vi "Process.vi"(8 "error in":errorcluster, 11 "Measurement.WavelengthSweeping.UI":refnum<class "Measurement.IVCurve.UI.lvclass">) -> (0 "error out":errorcluster, 3 "Measurement.WavelengthSweeping.UI out":refnum<class "Measurement.IVCurve.UI.lvclass">)   [LabVIEW 2017, in "Measurement.IVCurve.UI.lvclass"]
doc: "---------------------------------------------------------------\nJKI State Machine Objects™\nhttp://jki.net/state-machine-objects/\nCopyright (C) 2005-2015, JKI <info@jki.net>\nALL RIGHTS RESERVEDJKI State Machine Objects (SMO) 1.0.0.5\nJKI - JKI\nCopyright (c) 2016, JKI"
uses:
  Measurement.IVCurve.UI.lvclass
  D:/Program Files (x86)/National Instruments/LabVIEW 2017/vi.lib/JKI/JKI SMO/SMO/SMO.lvclass
  D:/Program Files (x86)/National Instruments/LabVIEW 2017/vi.lib/JKI/JKI SMO/SMO.UI/SMO.UI.lvclass
  <vilib>/JKI/JKI SMO/SMO/Typedefs/Parent Call--Enum.ctl
  Measurement.IVCurve/Typedefs/Measurement.IVCurve.Measured--Data.ctl
  Measurement.IVCurve/Measurement.IVCurve.lvclass
  D:/upwork/Laser Measurement Tool/Laser/project/Subsystems/Measurement/Measurement.lvclass
  Measurement.UI/Measurement.UI.lvclass
  <vilib>/JKI/JKI SMO/SMO/SMO.lvclass
  <vilib>/JKI/JKI SMO/SMO.UI/SMO.UI.lvclass
  Measurement/Measurement.lvclass
panel:
  in  "Clear Button":bool
  in  "Stop Button":bool
  in  "Pause Button":bool
  in  "Start Button":bool
  in  "Close Button":bool
  out "Initialized":bool
  out "I/V Curve":cluster{"X":dbl, "Y":dbl}[](graph) caption="XY Graph - Light"
  # "For instructions on how to use the JKI State Machine Objects, examples and video tutorials, visit:\nhttp://jki.net/state-machine-objects/\n\nJKI State Machine Objects™\nhttp://jki.net/state-machine-objects/\nCopyright (C) 2005-2015, JKI <info@jki.net>\nALL RIGHTS RESERVED"
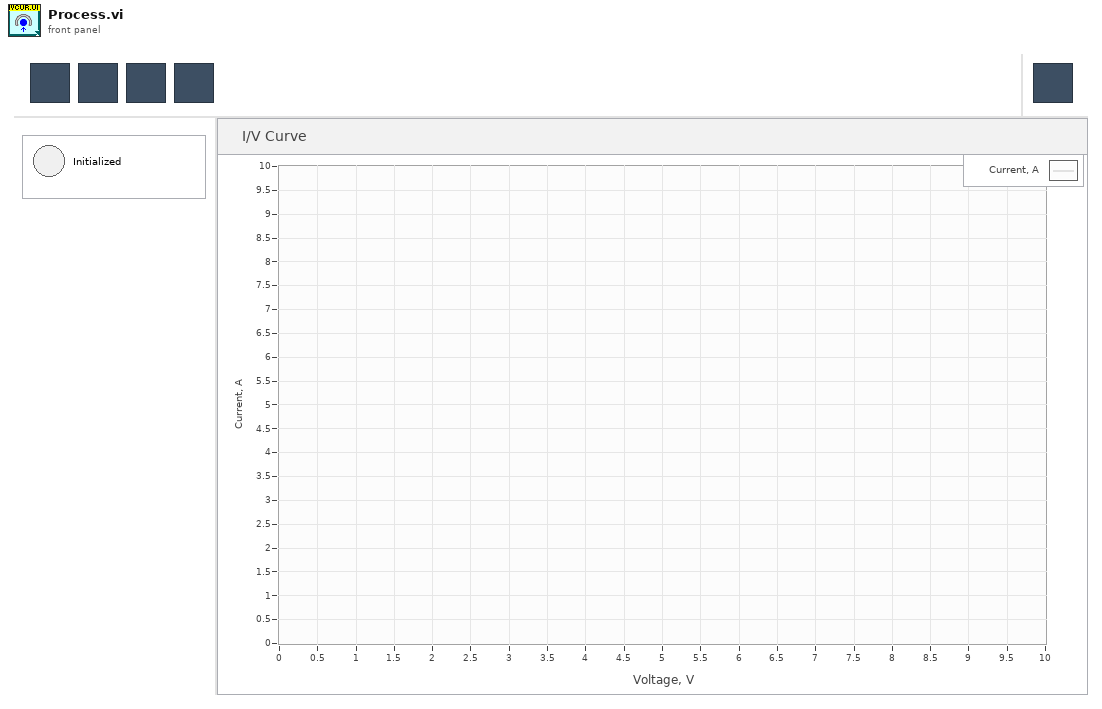
[diagram p1: front panel]
types:
  T1 = typedef "SMO.lvclass/Parent Call--Enum.ctl" = enum16{"Allows parent to run", "Does not request parent to run"}
  T2 = enum8{"Enabled", "Disabled", "Disabled and Grayed Out"}
  T3 = enum32{"invalid app kind", "Development System", "Run Time System", "Student Edition", "Embedded LabVIEW", "Evaluation", "Custom"}
  T4 = enum32{"Invalid", "Standard", "Closed", "Hidden", "Minimized", "Maximized"}
  T5 = typedef "Measurement.lvclass/PublicEvents--Measurement.Initialized.ctl" = bool
  T6 = typedef "Measurement.IVCurve.lvclass/Measurement.IVCurve.Measured--Data.ctl" = cluster{"Voltage, V":dbl, "Current, A":dbl}
  T7 = typedef "Measurement.lvclass/PublicEvents--Measurement.Measured.ctl" = variant
  T8 = typedef "Measurement.IVCurve.UI.lvclass/Dependencies--Cluster.ctl" = cluster{"Measurement.IVCurve":refnum<class "Measurement.IVCurve.lvclass">}
  T9 = cluster{"Core":cluster{"Current VI Reference":refnum<vi>, "Close Panel on Exit?":bool, "error":errorcluster}, "Self Reference":refnum<class "Measurement.IVCurve.UI.lvclass">, "Dependencies":T8, "IVCurve Data":cluster{"X":dbl, "Y":dbl}[]}
  T10 = typedef "Measurement.lvclass/PublicEvents--Measurement.Finished.ctl" = bool
  T11 = cluster{"Current VI Reference":refnum<vi>, "Close Panel on Exit?":bool, "error":errorcluster}
  T12 = typedef "SMO.lvclass/Protected Events.ctl" = cluster{"StopProcesses":refnum<user-event>, "AbortProcesses":refnum<user-event>, "Config Changed":refnum<user-event>, "Dependency":refnum<user-event>}
  T13 = cluster{"Event Registration Refnum":refnum<event-registration>, "Measurement Public Events":refnum<event-registration>}
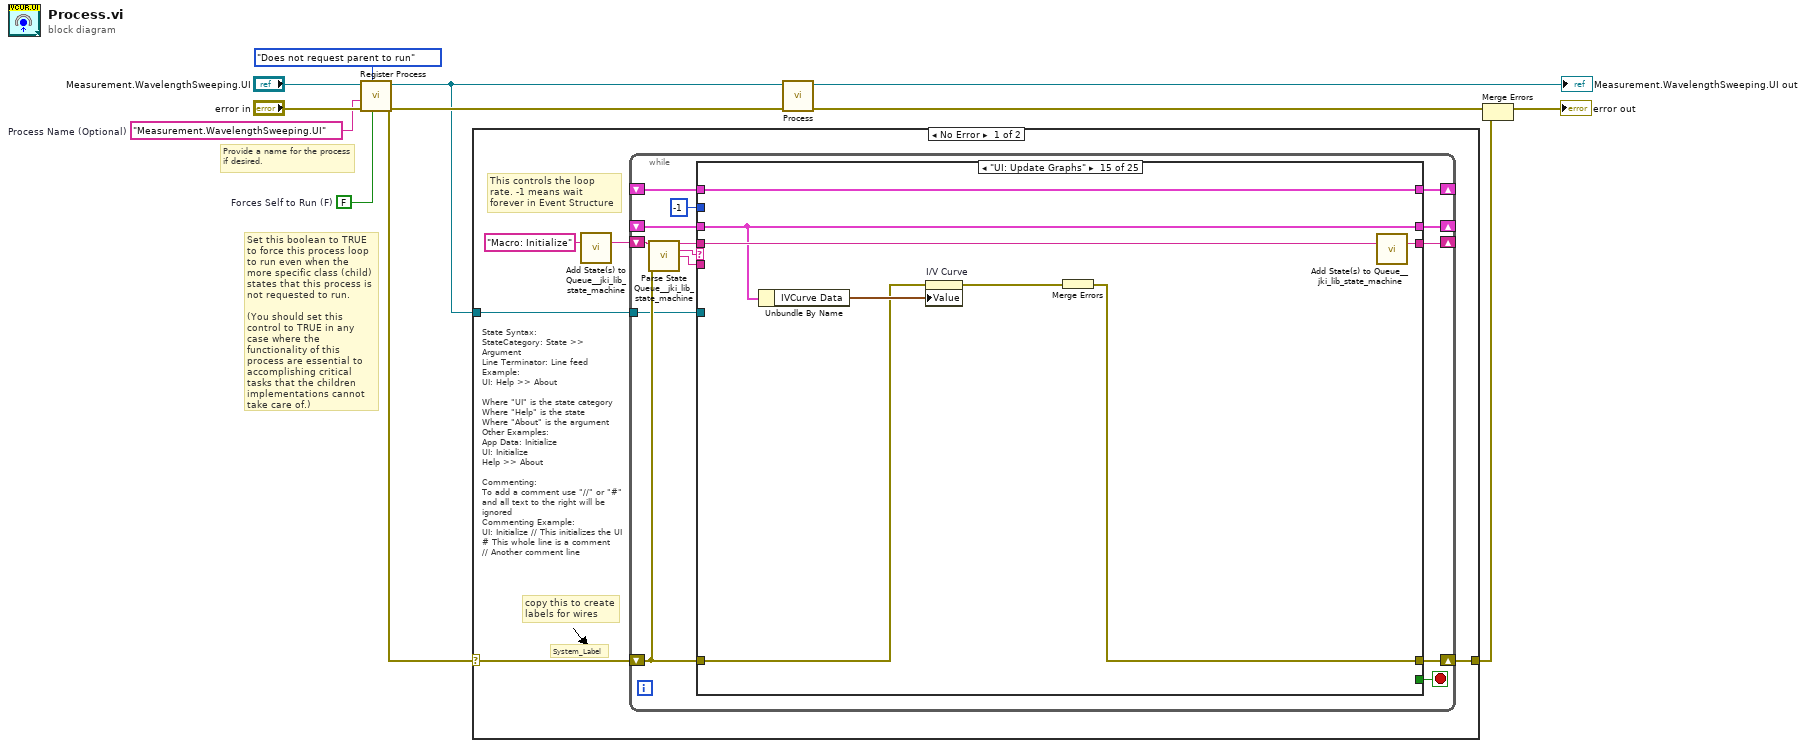
[diagram p0: block diagram]
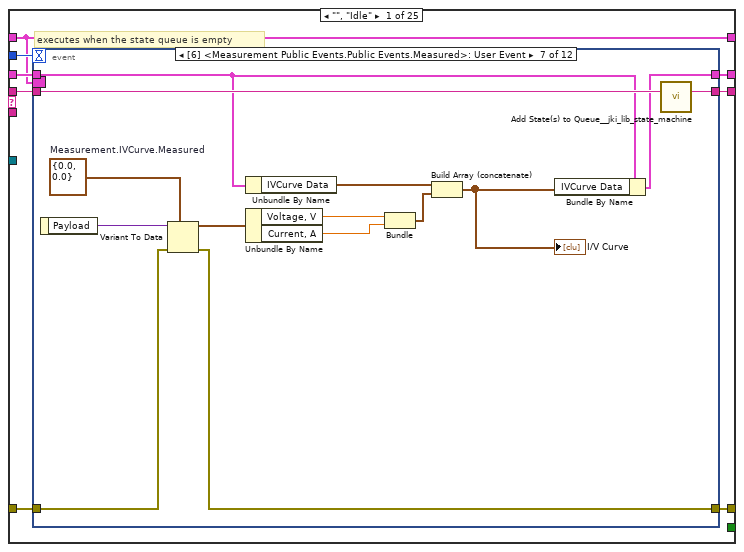
[diagram p2: hidden frame]
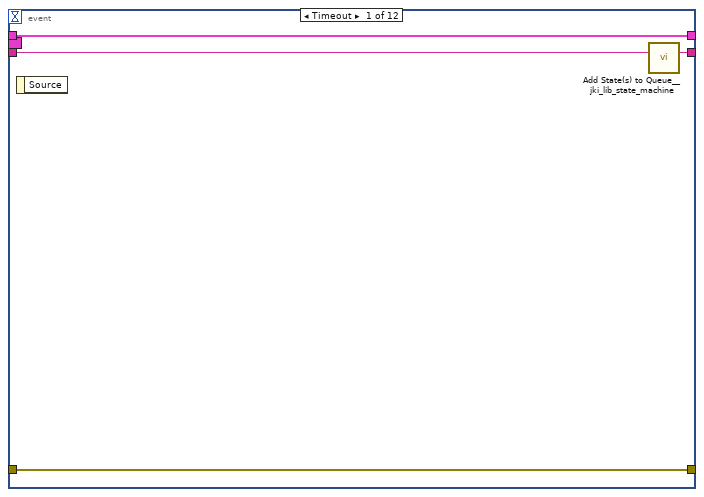
[diagram p3: hidden frame]
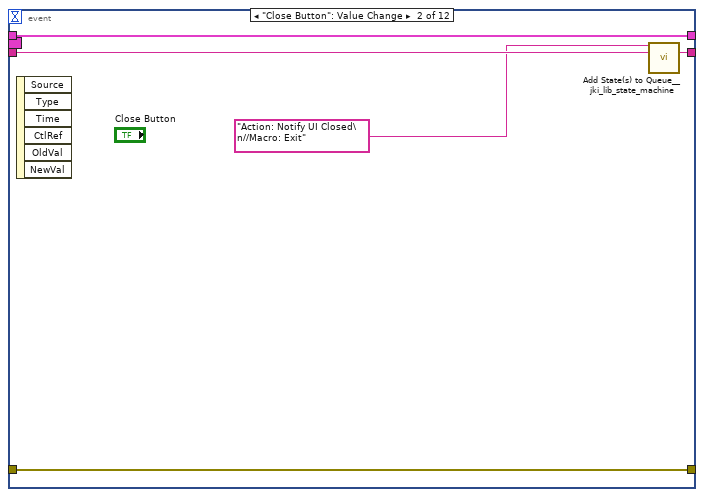
[diagram p4: hidden frame]
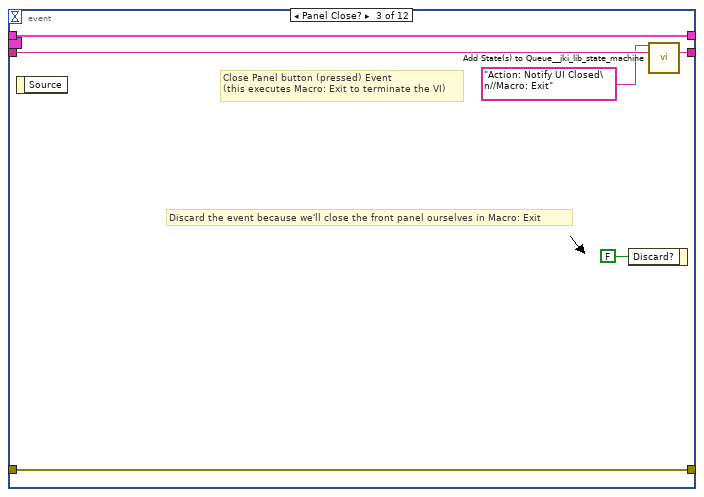
[diagram p5: hidden frame]
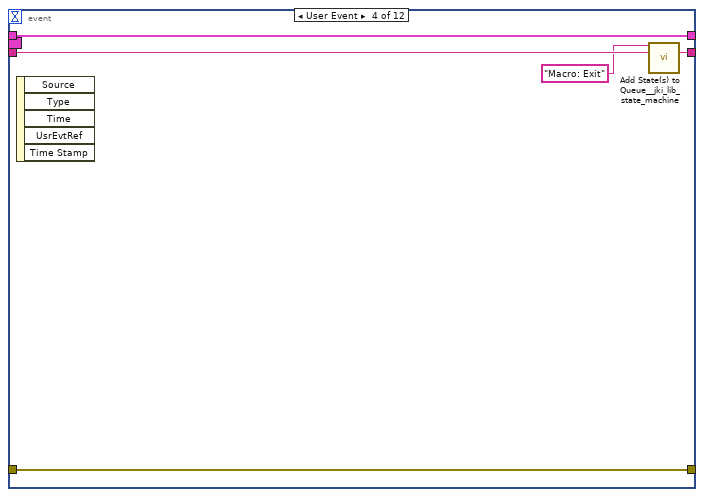
[diagram p6: hidden frame]
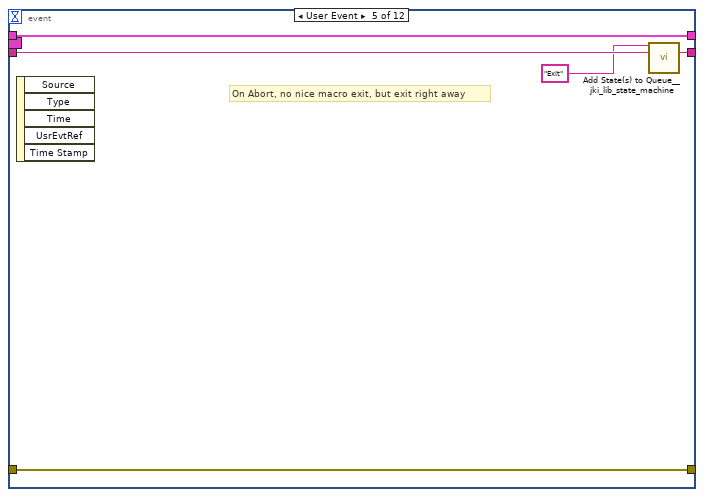
[diagram p7: hidden frame]
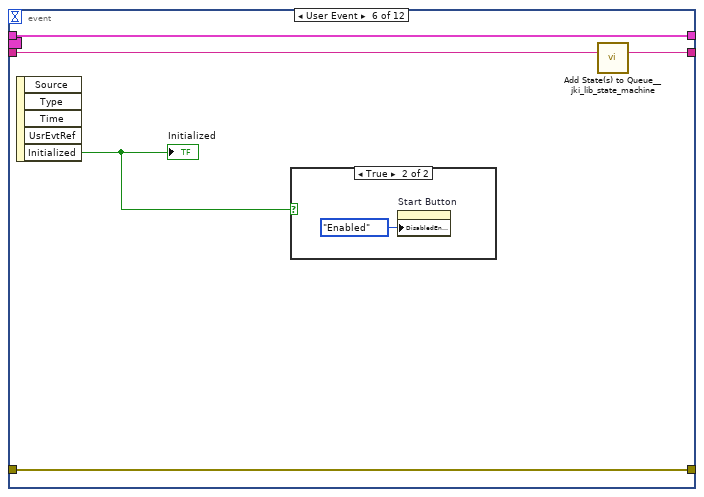
[diagram p8: hidden frame]
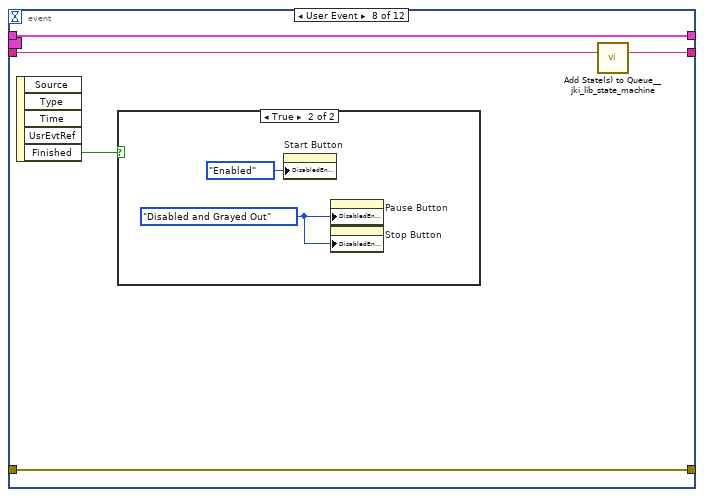
[diagram p10: hidden frame]
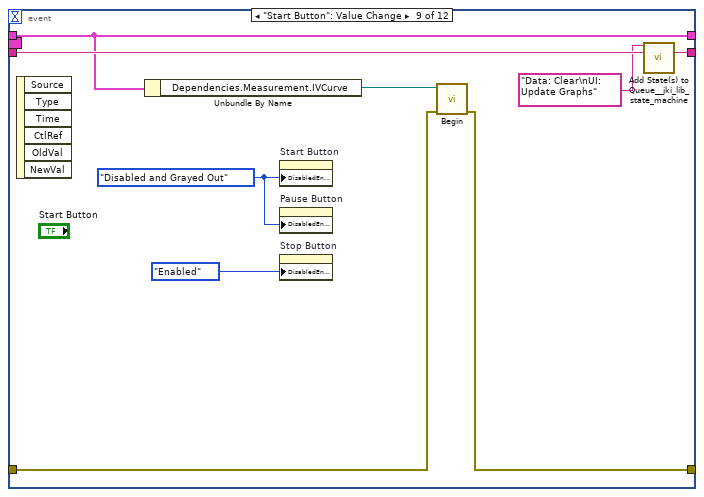
[diagram p12: hidden frame]
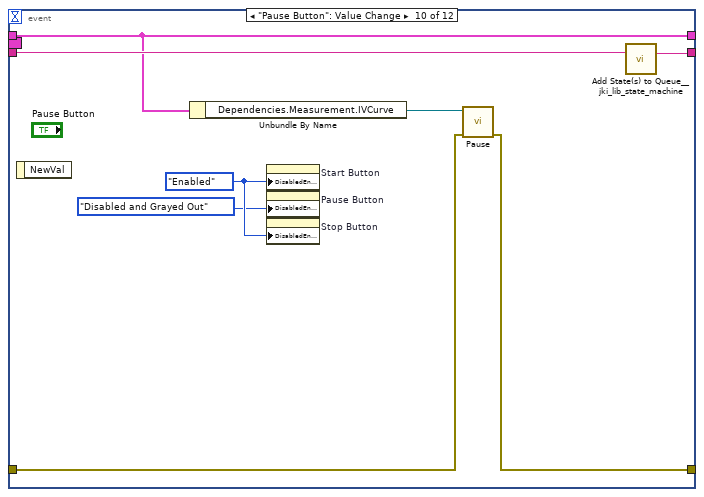
[diagram p13: hidden frame]
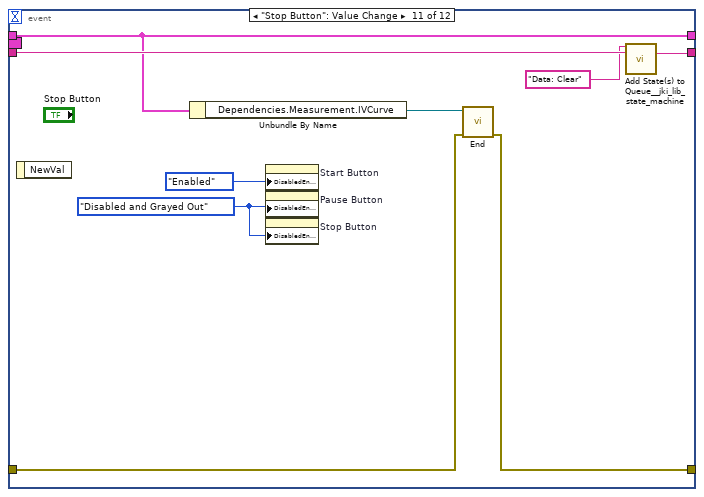
[diagram p14: hidden frame]
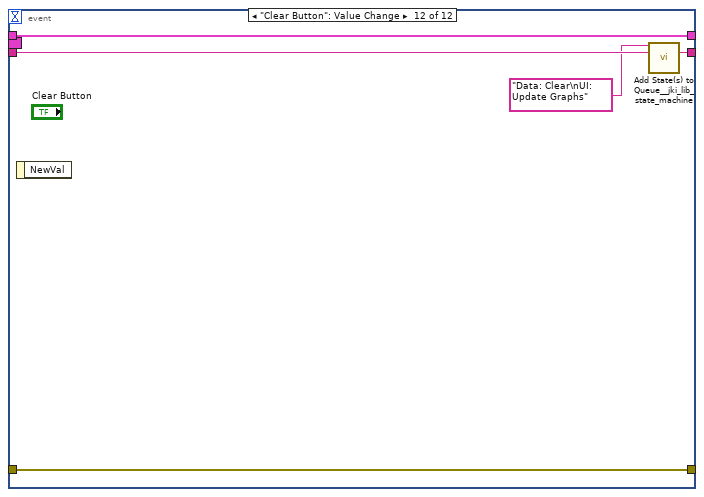
[diagram p15: hidden frame]
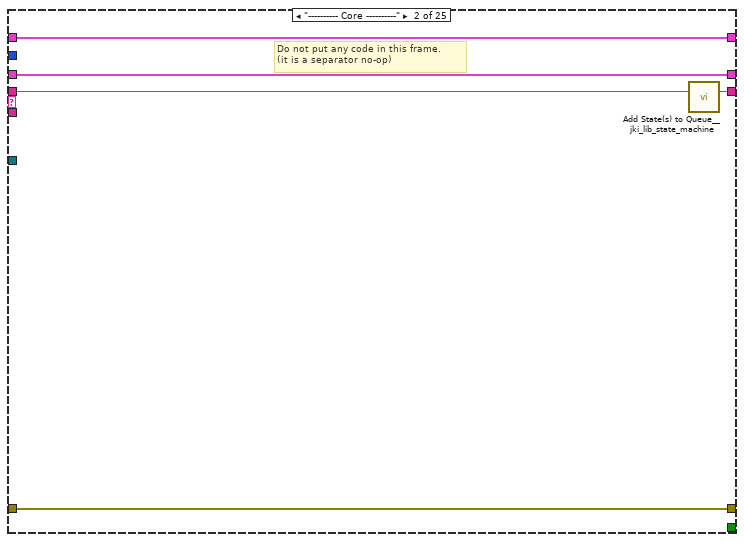
[diagram p16: hidden frame]
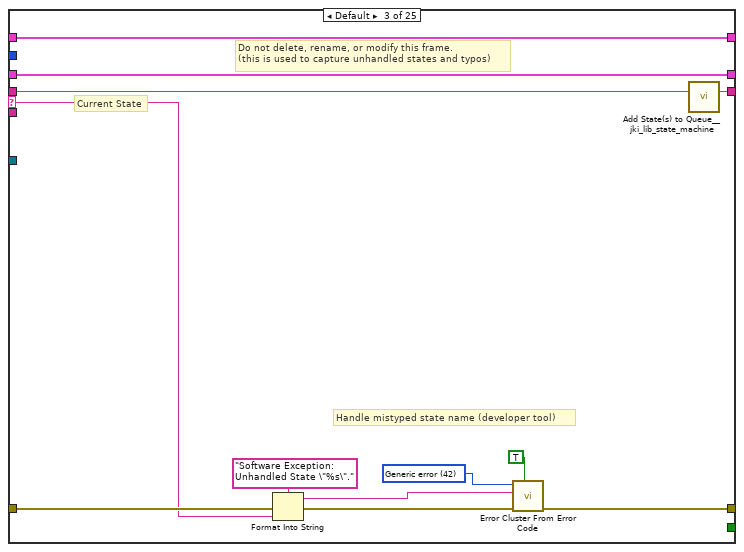
[diagram p17: hidden frame]
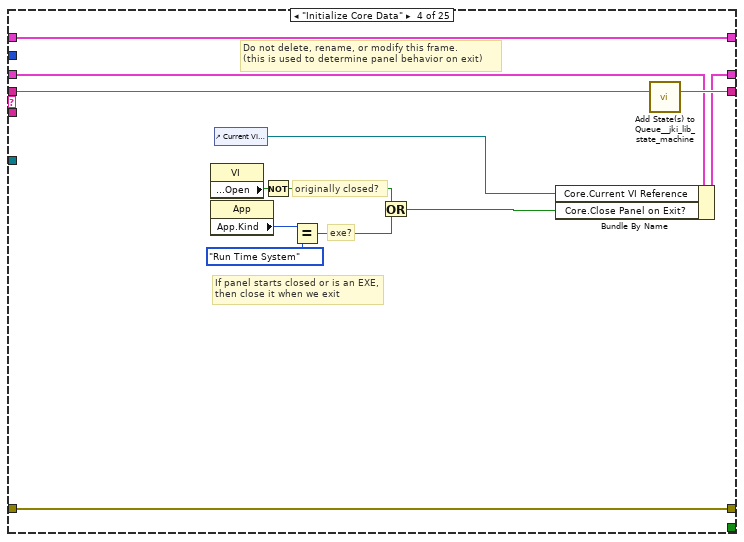
[diagram p18: hidden frame]
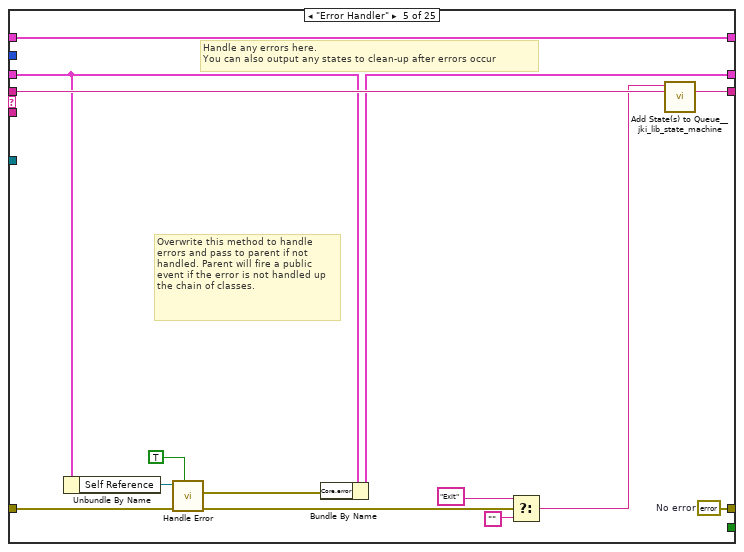
[diagram p19: hidden frame]
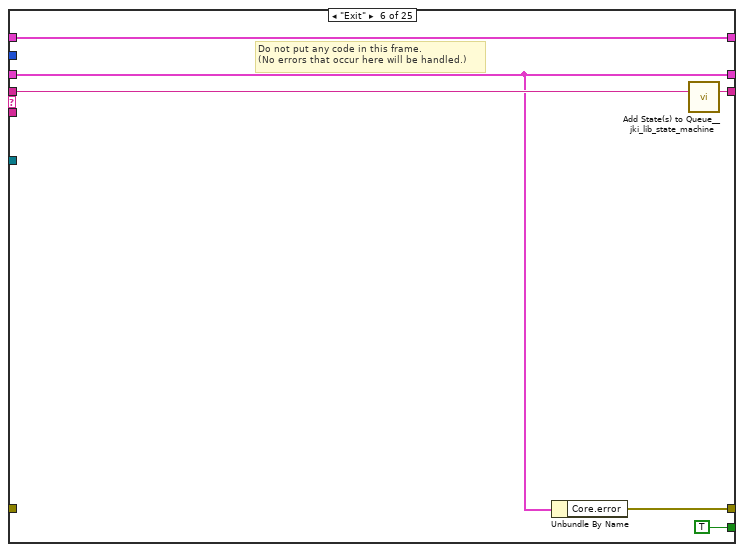
[diagram p20: hidden frame]
diagram:
  w2 = FALSE  # Forces Self to Run (F)
  w1 = "Measurement.WavelengthSweeping.UI"  # Process Name (Optional)
  # "Provide a name for the process\nif desired."
  # "Set this boolean to TRUE to force this process loop to run even when the more specific class (child) states that this process is not requested to run.\n\n(You should set this control to TRUE in any case where the functionality of this process are essential to accomplishing critical tasks that the children implementations cannot take care of.)"
  n1 = call <vilib>:"Register Process.vi"("Forces Self to Run (F)"=w2, "Parent Call"=Parent_Call--Enum."Does not request parent to run", "error in (no error)"="error in", "Process Name (optional)"=w1, "SMO"="Measurement.WavelengthSweeping.UI") -> ("error out"=w8:errorcluster, "SMO out"=w7:refnum<class "Measurement.IVCurve.UI.lvclass">)  [unwired: 5 in]
  n2 = case shown="No Error" w8 {
    selector: w8 -> [w13 w358]
    tunnel: w7 -> [w14 _]
    tunnel: [w12 w358] -> w4
    frame No Error {
      # "State Syntax:\nStateCategory: State >> Argument\nLine Terminator: Line feed\nExample:\nUI: Help >> About\n\nWhere \"UI\" is the state category\nWhere \"Help\" is the state\nWhere \"About\" is the argument\nOther Examples:\nApp Data: Initialize\nUI: Initialize\nHelp >> About\n\nCommenting:\nTo add a comment use \"//\" or \"#\" and all text to the right will be ignored\nCommenting Example:\nUI: Initialize // This initializes the UI\n# This whole line is a comment\n// Another comment line"
      # "copy this to create labels for wires"
      # "This controls the loop rate. -1 means wait forever in Event Structure"
      # "System_Label"
      n3 = call <vilib>:"Add State(s) to Queue__jki_lib_state_machine.vi"("State(s) in (\"\")"="Macro: Initialize") -> ("States Out"=w16:string)  [unwired: 14 in]
      n4 = while {
        shift-right: [w23] -> _
        shift-left: _ -> [w22]
        shift-right: [w26] -> w12
        shift-left: w13 -> [w20]
        shift-right: [w25] -> _
        shift-left: w16 -> [w27]
        tunnel: w14 -> [w19]
        shift-right: [w18] -> _
        shift-left: _ -> [w17]
        stop <- w24 stop-if-true
        n5 = call <vilib>:"Parse State Queue__jki_lib_state_machine.vi"("State Queue"=w27, "Error In (no error)"=w20) -> ("Remaining States"=w29:string, "Current State"=w30:string, "Arguments"=w28:string)  [unwired: 11 in]
        n6 = case shown="\"UI: Update Graphs\"" w30 {
          selector: w30 -> [_ _ w128 _ _ _ _ _ _ _ _ _ _ _ _ _ _ _ _ _ _ _ _ _ _]
          tunnel: w29 -> [w38 w126 w132 w151 w165 w171 w176 w189 w194 w203 w208 w216 w223 w239 w274 w279 w288 w302 w307 w318 w323 w337 w343 w350 w357]
          tunnel: w28 -> [_ _ _ _ _ _ _ _ _ _ _ _ w217 w233 _ _ _ _ _ _ _ _ _ _ _]
          tunnel: w22 -> [w36 w123 w130 w142 w154 w167 w173 _ w193 w198 w205 w214 w221 w235 w271 w276 w284 w293 w304 w315 w320 w329 w341 w346 w353]
          tunnel: [w35 w124 w134 w148 w156 w166 w174 w178 w191 w199 w206 w209 w218 w236 w268 w277 w286 w300 w305 w309 w321 w331 w338 w347 w351] -> w26
          tunnel: w20 -> [w34 w124 w133 w148 w161 _ w174 w186 w191 w200 w206 w212 w219 w237 w267 w277 w286 w300 w305 w310 w321 w333 w339 w347 w352]
          tunnel: [w37 w125 w131 w150 w164 w170 w175 w188 w195 w202 w207 w215 w222 w238 w273 w278 w287 w301 w306 w317 w322 w336 w342 w349 w356] -> w25
          tunnel: [_ _ _ _ _ TRUE _ _ _ _ _ _ _ _ _ _ _ _ _ _ _ _ _ _ _] -> w24
          tunnel: [w33 w123 w130 w149 w153 w167 w173 w187 w192 w198 w205 w214 w221 w235 w271 w276 w284 w293 w304 w315 w320 w329 w341 w345 w353] -> w23
          tunnel: -1 ("Timeout") -> [w32 _ _ _ _ _ _ _ _ _ _ _ _ _ _ _ _ _ _ _ _ _ _ _ _]
          tunnel: w19 -> [_ _ _ _ _ _ _ w184 _ _ _ _ _ _ _ _ _ _ _ _ _ _ _ _ _]
          tunnel: [w31 w122 w127 w139 w163 w168 w172 w183 w196 w197 w204 w213 w220 w232 w272 w275 w285 w294 w303 w316 w319 w326 w340 w348 w355] -> w18
          tunnel: w17 -> [w31 w122 w127 w139 w163 w168 w172 w183 w196 w197 w204 w213 w220 w232 w272 w275 w285 w294 w303 w316 w319 _ w340 w348 w355]
          frame "", "Idle" {
            # "executes when the state queue is empty"
            n7 = event shown="[6] <Measurement Public Events.Public Events.Measured>: User Event" {
              selector: w31 -> [_ _ _ _ _ _ _ _ _ _ _ _]
              dyn-events: _ -> [_ _ _ _ _ _ _ _ _ _ _ _]
              timeout: w32 -> [_ _ _ _ _ _ _ _ _ _ _ _]
              tunnel: w38 -> [w42 w47 w53 w58 w63 w65 w82 w85 w98 w106 w115 w121]
              tunnel: [w41 w46 w52 w57 w62 w66 w83 w86 w99 w107 w116 w120] -> w37
              tunnel: w36 -> [w39 w44 w49 w55 w60 w67 w75 w87 w97 w105 w114 w118]
              tunnel: [w40 w45 w48 w56 w61 w68 w80 w88 w94 w102 w111 w119] -> w35
              tunnel: w34 -> [w40 w45 w48 w56 w61 w68 w81 w88 w95 w103 w112 w119]
              tunnel: [w39 w44 w49 w55 w60 w67 w74 w87 w97 w105 w114 w118] -> w33
              event Timeout {
                n8 = event-data() -> ()  [unwired: 1 in, 1 out]
                n9 = call <vilib>:"Add State(s) to Queue__jki_lib_state_machine.vi"("State(s) in (\"\")"=w42) -> ("States Out"=w41:string)  [unwired: 14 in]
              }
              event "Close Button": Value Change {
                n10 = event-data() -> ()  [unwired: 1 in, 6 out]
                n11 = call <vilib>:"Add State(s) to Queue__jki_lib_state_machine.vi"("State(s) in Front (\"\")"="Action: Notify UI Closed\n//Macro: Exit" ("State(s) in Front (\"\")"), "State(s) in (\"\")"=w47) -> ("States Out"=w46:string)  [unwired: 13 in]
              }
              event Panel Close? {
                # "Discard the event because we'll close the front panel ourselves in Macro: Exit"
                # "Close Panel button (pressed) Event\n(this executes Macro: Exit to terminate the VI)"
                n12 = event-data() -> ()  [unwired: 1 in, 1 out]
                n13 = event-data("Discard?"=FALSE) -> ()  [unwired: 1 in, 1 out]
                n14 = call <vilib>:"Add State(s) to Queue__jki_lib_state_machine.vi"("State(s) in Front (\"\")"="Action: Notify UI Closed\n//Macro: Exit", "State(s) in (\"\")"=w53) -> ("States Out"=w52:string)  [unwired: 13 in]
              }
              event User Event {
                n15 = event-data() -> ()  [unwired: 1 in, 5 out]
                n16 = call <vilib>:"Add State(s) to Queue__jki_lib_state_machine.vi"("State(s) in Front (\"\")"="Macro: Exit", "State(s) in (\"\")"=w58) -> ("States Out"=w57:string)  [unwired: 13 in]
              }
              event User Event {
                # "On Abort, no nice macro exit, but exit right away"
                n17 = event-data() -> ()  [unwired: 1 in, 5 out]
                n18 = call <vilib>:"Add State(s) to Queue__jki_lib_state_machine.vi"("State(s) in Front (\"\")"="Exit", "State(s) in (\"\")"=w63) -> ("States Out"=w62:string)  [unwired: 13 in]
              }
              event User Event {
                n19 = event-data() -> ("Initialized"=w64:T5)  [unwired: 1 in, 4 out]
                "Initialized" <- w64
                n20 = case shown="True" w64 {
                  frame False {
                  }
                  frame True {
                    n21 = property on="Start Button" class="Bool"("DisabledEnum"=T2."Enabled" ("Disabled")) -> ()  [unwired: 2 in, 2 out]
                  }
                }
                n22 = call <vilib>:"Add State(s) to Queue__jki_lib_state_machine.vi"("State(s) in (\"\")"=w65) -> ("States Out"=w66:string)  [unwired: 14 in]
              }
              event User Event {
                w71 = T6 {"Voltage, V"=0.0, "Current, A"=0.0}  # Measurement.IVCurve.Measured
                n23 = event-data() -> ("Payload"=w72:T7)  [unwired: 1 in]
                n24 = Variant To Data(error in=w81, type=w71, Variant=w72) -> (data=w70:T6, error out=w80:errorcluster)
                n25 = Unbundle By Name(w75) -> ("IVCurve Data"=w77:cluster{"X":dbl, "Y":dbl}[])
                n26 = Unbundle By Name(w70) -> ("Voltage, V"=w79:dbl, "Current, A"=w78:dbl)
                n27 = Bundle("Voltage, V"=w79, "Current, A"=w78) -> (w76:cluster{"Voltage, V":dbl, "Current, A":dbl})  [unwired: 1 in]
                n28 = Build Array (concatenate)(w77, w76) -> (w73:cluster{"Voltage, V":dbl, "Current, A":dbl}[])
                "I/V Curve" <- w73
                n29 = Bundle By Name(cluster=w75, "IVCurve Data"=w73) -> (w74:T9)
                n30 = call <vilib>:"Add State(s) to Queue__jki_lib_state_machine.vi"("State(s) in (\"\")"=w82) -> ("States Out"=w83:string)  [unwired: 14 in]
              }
              event User Event {
                n31 = event-data() -> ("Finished"=w84:T10)  [unwired: 1 in, 4 out]
                n32 = case shown="True" w84 {
                  frame False {
                  }
                  frame True {
                    w89 = T2."Disabled and Grayed Out" ("Disabled")
                    n33 = property on="Start Button" class="Bool"("DisabledEnum"=T2."Enabled" ("Disabled")) -> ()  [unwired: 2 in, 2 out]
                    n34 = property on="Pause Button" class="Bool"("DisabledEnum"=w89) -> ()  [unwired: 2 in, 2 out]
                    n35 = property on="Stop Button" class="Bool"("DisabledEnum"=w89) -> ()  [unwired: 2 in, 2 out]
                  }
                }
                n36 = call <vilib>:"Add State(s) to Queue__jki_lib_state_machine.vi"("State(s) in (\"\")"=w85) -> ("States Out"=w86:string)  [unwired: 14 in]
              }
              event "Start Button": Value Change {
                w92 = T2."Disabled and Grayed Out" ("Disabled")
                n37 = event-data() -> ()  [unwired: 1 in, 6 out]
                n38 = Unbundle By Name(w97) -> ("Dependencies.Measurement.IVCurve"=w96:refnum<class "Measurement.IVCurve.lvclass">)
                n39 = property on="Start Button" class="Bool"("DisabledEnum"=w92) -> ()  [unwired: 2 in, 2 out]
                n40 = property on="Pause Button" class="Bool"("DisabledEnum"=w92) -> ()  [unwired: 2 in, 2 out]
                n41 = property on="Stop Button" class="Bool"("DisabledEnum"=T2."Enabled" ("Disabled")) -> ()  [unwired: 2 in, 2 out]
                n42 = call "Begin.vi"("error in (no error)"=w95, "Measurement in"=w96) -> ("error out"=w94:errorcluster)  [unwired: 8 in, 1 out]
                n43 = call <vilib>:"Add State(s) to Queue__jki_lib_state_machine.vi"("State(s) in Front (\"\")"="Data: Clear\nUI: Update Graphs", "State(s) in (\"\")"=w98) -> ("States Out"=w99:string)  [unwired: 13 in]
              }
              event "Pause Button": Value Change {
                w101 = T2."Enabled" ("Disabled")
                n44 = event-data() -> ()  [unwired: 1 in, 1 out]
                n45 = Unbundle By Name(w105) -> ("Dependencies.Measurement.IVCurve"=w104:refnum<class "Measurement.IVCurve.lvclass">)
                n46 = property on="Start Button" class="Bool"("DisabledEnum"=w101) -> ()  [unwired: 2 in, 2 out]
                n47 = property on="Pause Button" class="Bool"("DisabledEnum"=T2."Disabled and Grayed Out" ("Disabled")) -> ()  [unwired: 2 in, 2 out]
                n48 = property on="Stop Button" class="Bool"("DisabledEnum"=w101) -> ()  [unwired: 2 in, 2 out]
                n49 = call "Pause.vi"("error in (no error)"=w103, "Measurement in"=w104) -> ("error out"=w102:errorcluster)  [unwired: 8 in, 1 out]
                n50 = call <vilib>:"Add State(s) to Queue__jki_lib_state_machine.vi"("State(s) in (\"\")"=w106) -> ("States Out"=w107:string)  [unwired: 14 in]
              }
              event "Stop Button": Value Change {
                w109 = T2."Disabled and Grayed Out" ("Disabled")
                n51 = event-data() -> ()  [unwired: 1 in, 1 out]
                n52 = Unbundle By Name(w114) -> ("Dependencies.Measurement.IVCurve"=w113:refnum<class "Measurement.IVCurve.lvclass">)
                n53 = property on="Start Button" class="Bool"("DisabledEnum"=T2."Enabled" ("Disabled")) -> ()  [unwired: 2 in, 2 out]
                n54 = property on="Pause Button" class="Bool"("DisabledEnum"=w109) -> ()  [unwired: 2 in, 2 out]
                n55 = property on="Stop Button" class="Bool"("DisabledEnum"=w109) -> ()  [unwired: 2 in, 2 out]
                n56 = call "End.vi"("error in (no error)"=w112, "Measurement in"=w113) -> ("error out"=w111:errorcluster)  [unwired: 8 in, 1 out]
                n57 = call <vilib>:"Add State(s) to Queue__jki_lib_state_machine.vi"("State(s) in Front (\"\")"="Data: Clear", "State(s) in (\"\")"=w115) -> ("States Out"=w116:string)  [unwired: 13 in]
              }
              event "Clear Button": Value Change {
                n58 = event-data() -> ()  [unwired: 1 in, 1 out]
                n59 = call <vilib>:"Add State(s) to Queue__jki_lib_state_machine.vi"("State(s) in Front (\"\")"="Data: Clear\nUI: Update Graphs", "State(s) in (\"\")"=w121) -> ("States Out"=w120:string)  [unwired: 13 in]
              }
            }
          }
          frame "---------- Core ----------" {
            # "Do not put any code in this frame.\n(it is a separator no-op)"
            n60 = call <vilib>:"Add State(s) to Queue__jki_lib_state_machine.vi"("State(s) in (\"\")"=w126) -> ("States Out"=w125:string)  [unwired: 14 in]
          }
          frame Default {
            w137 = 42 items=["No error", "Argument error", "Memory is full", "Out of zone", "End of file", "File already open", "Generic file I/O error", "File not found", "File permission error", "Disk is full", "Duplicate path", "Too many files open", "System feature not enabled", "Resource file not found", "Cannot add resource", "Resource not found", "Image not found", "Image memory error", "Pen does not exist", "Config type invalid", "Config token not found", "Config parse error", "Config memory error", "Bad external code format", "Bad external code offset", "External code not present", "Null window", "Destroy window error", "Null menu", "Print aborted", "Bad print record", "Print driver error", "Windows error during printing", "Memory error during printing", "Print dialog error", "Generic print error", "Invalid device refnum", "Device not found", "Device parameter error", "Device unit error", "Cannot open device", "Device call aborted", "Generic error", "Cancelled by user", "Object ID too low", "Object ID too high", "Object not in heap", "Unknown heap", "Unknown object (invalid DefProc)", "Unknown object (DefProc not in table)", "Message out of range", "Invalid (null) method", "Unknown message", "Manager call not supported", "Bad address", "Network operation in progress", "Network operation timed out", "Connection is busy", "Network attribute not supported", "Network error", "Address in use", "System out of memory", "Connection aborted", "Connection refused", "Not connected", "Already connected", "Connection closed", "Initialization error (interapplication manager)", "Bad occurrence", "Wait on unbound occurrence handler", "Occurrence queue overflow", "Datalog type conflict", "Unused", "Unrecognized type (interapplication manager)", "Memory corrupt", "Failed to make temporary DLL", "Old CIN version", "Drag socket not found", "Failed to load drop-object", "Failed to register OLE object", "Failed to release OLE object", "Format specifier type mismatch", "Unknown format specifier", "Too few format specifiers", "Too many format specifiers", "Scan failed", "Newer CIN version", "Error converting to variant", "Runtime menu error", "Password tampered", "Variant attribute not found", "Incompatible variant data type", "Event data is not available", "Event Store is not present", "Occurrence is not found", "Event Queue is not created", "Event info is not available", "Refnum passed is NULL", "Error retrieving Class GUID", "Error retrieving CoClass GUID", "Error retrieving TypeLib GUID.", "Bad built application magic bytes.", "Specific driver is different from the specific driver associated with the Logical Name.", "There is no session opened to the class driver.", "Max Error", "MAX - Error with config objects", "MAX - Error loading configuration", "MAX - Group not supported"]
            # "Current State"
            # "Do not delete, rename, or modify this frame.\n(this is used to capture unhandled states and typos)"
            # "Handle mistyped state name (developer tool)"
            n61 = Format Into String(format string="Software Exception: Unhandled State \"%s\"." ("message"), error in=w133, w128) -> (resulting string=w136:string, error out=w135:errorcluster)  [unwired: 1 in]
            n62 = call <vilib>:"Error Cluster From Error Code.vi"("show call chain? (False)"=TRUE, "error in (no error)"=w135, "error message (\"\")"=w136, "error code (0)"=w137) -> ("error out"=w134:errorcluster)  [unwired: 5 in]
            n63 = call <vilib>:"Add State(s) to Queue__jki_lib_state_machine.vi"("State(s) in (\"\")"=w132) -> ("States Out"=w131:string)  [unwired: 14 in]
          }
          frame "Initialize Core Data" {
            # "Do not delete, rename, or modify this frame.\n(this is used to determine panel behavior on exit)"
            # "originally closed?"
            # "exe?"
            # "If panel starts closed or is an EXE, then close it when we exit"
            n64 = property class="VI"() -> ("Front Panel.Open"=w147:bool)  [unwired: 2 in, 2 out]
            n65 = property class="App"() -> ("App.Kind"=w146:T3)  [unwired: 2 in, 2 out]
            n66 = control-ref of="Current VI Reference"() -> (w140:refnum<vi>)
            n67 = Not(x=w147) -> (.not. x?=w144:bool)
            n68 = Equal?(x=w146, y=T3."Run Time System" ("Application:Kind")) -> (x = y?=w143:bool)
            n69 = Or(x=w144, y=w143) -> (x .or. y?=w141:bool)
            n70 = Bundle By Name(cluster=w142, "Core.Current VI Reference"=w140, "Core.Close Panel on Exit?"=w141) -> (w149:T9)
            n71 = call <vilib>:"Add State(s) to Queue__jki_lib_state_machine.vi"("State(s) in (\"\")"=w151) -> ("States Out"=w150:string)  [unwired: 14 in]
          }
          frame "Error Handler" {
            w156 = errorcluster {"status"=FALSE, "code"=0, "source"=""}  # No error
            # "Overwrite this method to handle errors and pass to parent if not handled. Parent will fire a public event if the error is not handled up the chain of classes."
            # "Handle any errors here.\nYou can also output any states to clean-up after errors occur"
            n72 = Unbundle By Name(w154) -> ("Self Reference"=w162:refnum<class "Measurement.IVCurve.UI.lvclass">)
            n73 = call-dynamic "Handle Error.vi"("Stop on Unhandled Error (T)"=TRUE, "error in"=w161, "SMO"=w162) -> ("handling error"=w157:errorcluster, "Unhandled error"=w155:errorcluster)  [unwired: 6 in, 1 out]
            n74 = Bundle By Name(cluster=w154, "Core.error"=w155) -> (w153:T9)
            n75 = Select(t="Exit", s=w157, f="") -> (s? t:f=w158:string)
            n76 = call <vilib>:"Add State(s) to Queue__jki_lib_state_machine.vi"("State(s) in Front (\"\")"=w158, "State(s) in (\"\")"=w165) -> ("States Out"=w164:string)  [unwired: 13 in]
          }
          frame "Exit" {
            # "Do not put any code in this frame.\n(No errors that occur here will be handled.)"
            n77 = Unbundle By Name(w167) -> ("Core.error"=w166:errorcluster)
            n78 = call <vilib>:"Add State(s) to Queue__jki_lib_state_machine.vi"("State(s) in (\"\")"=w171) -> ("States Out"=w170:string)  [unwired: 14 in]
          }
          frame "---------- Data ----------" {
            # "Do not put any code in this frame.\n(It is a separator no-op. You can make a copy of this frame to create a new Data frame)"
            n79 = call <vilib>:"Add State(s) to Queue__jki_lib_state_machine.vi"("State(s) in (\"\")"=w176) -> ("States Out"=w175:string)  [unwired: 14 in]
          }
          frame "Data: Initialize" {
            w177 = cluster{"X":dbl, "Y":dbl}[] []  # IVCurve Data
            w182 = T11 {"Current VI Reference"=refnum, "Close Panel on Exit?"=FALSE, "error"={"status"=FALSE, "code"=0, "source"=""}}  # Core
            w185 = refnum<class "Measurement.IVCurve.UI.lvclass"> refnum  # Self Reference
            # "do not delete - used by framework"
            # "Data names and types of shift register data are defined by this bundle."
            # "Initialize the shift-register data, here.\n(data names are defined by what you wire into the bundle function)"
            n80 = Variant To Data(error in=w186, type=w185, Variant=w184) -> (data=w181:refnum<class "Measurement.IVCurve.UI.lvclass">, error out=w179:errorcluster)
            n81 = call "Measurement.IVCurve.UI.GetDependencies.vi"("error in (no error)"=w179, "Measurement.IVCurve.UI in"=w181) -> ("error out"=w178:errorcluster, "Dependencies"=w180:T8)  [unwired: 7 in, 1 out]
            n82 = Bundle("Core"=w182, "Self Reference"=w181, "Dependencies"=w180, "IVCurve Data"=w177) -> (w187:T9)  [unwired: 1 in]
            n83 = call <vilib>:"Add State(s) to Queue__jki_lib_state_machine.vi"("State(s) in (\"\")"=w189) -> ("States Out"=w188:string)  [unwired: 14 in]
          }
          frame "Data: Clear" {
            n84 = Bundle By Name(cluster=w193, "IVCurve Data"=cluster{"X":dbl, "Y":dbl}[] [] ("SMU Data")) -> (w192:T9)
            n85 = call <vilib>:"Add State(s) to Queue__jki_lib_state_machine.vi"("State(s) in (\"\")"=w194) -> ("States Out"=w195:string)  [unwired: 14 in]
          }
          frame "Data: Cleanup" {
            # "Cleanup any data and references, here.\n(this is called automatically, by the Macro: Exit)"
            n86 = Unbundle By Name(w198) -> ("Core.Current VI Reference"=w201:refnum<vi>)
            n87 = Close Reference(reference=w201, error in (no error)=w200) -> (error out=w199:errorcluster)
            n88 = call <vilib>:"Add State(s) to Queue__jki_lib_state_machine.vi"("State(s) in (\"\")"=w203) -> ("States Out"=w202:string)  [unwired: 14 in]
          }
          frame "---------- UI ----------" {
            # "Do not put any code in this frame.\n(It is a separator no-op. You can make a copy of this frame to create a new UI frame)"
            n89 = call <vilib>:"Add State(s) to Queue__jki_lib_state_machine.vi"("State(s) in (\"\")"=w208) -> ("States Out"=w207:string)  [unwired: 14 in]
          }
          frame "UI: Initialize" {
            w211 = T2."Disabled and Grayed Out" ("Disabled")
            # "Initialize the User Interface, here.\n(this is called automatically, by the Macro: Init)"
            n90 = invoke on="Initialized" class="Bool (strict)" method="Reinit To Default"(error in=w212) -> (error out=w210:errorcluster)  [unwired: 2 in, 2 out]
            n91 = property on="Start Button" class="Bool"("DisabledEnum"=w211) -> ()  [unwired: 2 in, 2 out]
            n92 = property on="Pause Button" class="Bool"("DisabledEnum"=w211) -> ()  [unwired: 2 in, 2 out]
            n93 = property on="Stop Button" class="Bool"("DisabledEnum"=w211) -> ()  [unwired: 2 in, 2 out]
            n94 = invoke on="I/V Curve" class="XYGraph (strict)" method="Reinit To Default"(error in=w210) -> (error out=w209:errorcluster)  [unwired: 2 in, 2 out]
            n95 = call <vilib>:"Add State(s) to Queue__jki_lib_state_machine.vi"("State(s) in (\"\")"=w216) -> ("States Out"=w215:string)  [unwired: 14 in]
          }
          frame "UI: Cursor Set" {
            # "Argument"
            # "Initialize the User Interface, here.\n(this is called automatically, by the Macro: Init)"
            n96 = disable-structure shown="Default" {
              disable-tunnel: w219 -> [w224 w227]
              disable-tunnel: [w224 w226] -> w218
              disable-tunnel: w217 -> [_ w225]
              frame condition #0 {
              }
              frame condition #1 (active) {
                n97 = case shown="\"Idle\", Default" w225 {
                  tunnel: w227 -> [w229 w231]
                  tunnel: [w228 w230] -> w226
                  frame "Idle", Default {
                    n98 = call <vilib>:"Unset Busy.vi"("error in (no error)"=w229) -> ("error out"=w228:errorcluster)  [unwired: 10 in]
                  }
                  frame "Busy" {
                    n99 = call <vilib>:"Set Busy.vi"("error in (no error)"=w231) -> ("error out"=w230:errorcluster)  [unwired: 9 in, 1 out]
                  }
                }
              }
            }
            n100 = call <vilib>:"Add State(s) to Queue__jki_lib_state_machine.vi"("State(s) in (\"\")"=w223) -> ("States Out"=w222:string)  [unwired: 14 in]
          }
          frame "UI: Front Panel State" {
            # "Argument"
            # "Set Front Panel Open or Closed\n(Usage: \"UI: Front Panel State >> Open|Close\")"
            n101 = Unbundle By Name(w235) -> ("Core.Current VI Reference"=w234:refnum<vi>)
            n102 = disable-structure shown="Default" {
              disable-tunnel: w237 -> [w243 w266]
              disable-tunnel: [w242 w266] -> w236
              disable-tunnel: w234 -> [w241 _]
              disable-tunnel: w233 -> [w240 _]
              frame condition #0 (active) {
                n103 = case shown="\"Close\"" w240 {
                  tunnel: w243 -> [w247 w260]
                  tunnel: [w249 w261] -> w242
                  tunnel: w241 -> [w248 w258]
                  frame "Open", Default {
                    n104 = property class="VI"(reference=w248, error in=w247) -> (reference out=w245:refnum<vi>, error out=w246:errorcluster, "FP.State"=w244:T4)
                    n105 = case shown="\"Closed\"" w244 {
                      tunnel: [w252 w255] -> w249
                      tunnel: w246 -> [w251 w255]
                      tunnel: w245 -> [w250 _]
                      frame "Closed" {
                        n106 = invoke class="VI" method="FP.Open"(reference=w250, error in=w251, "Activate"=TRUE, "State"=T4."Standard") -> (error out=w252:errorcluster)  [unwired: 1 in, 4 out]
                      }
                      frame Default {
                      }
                    }
                  }
                  frame "Close" {
                    n107 = property class="VI"(reference=w258, error in=w260) -> (reference out=w257:refnum<vi>, error out=w259:errorcluster, "FP.State"=w256:T4)
                    n108 = case shown="Default" w256 {
                      tunnel: [w262 w265] -> w261
                      tunnel: w259 -> [w262 w264]
                      tunnel: w257 -> [_ w263]
                      frame "Invalid", "Closed" {
                      }
                      frame Default {
                        n109 = invoke class="VI" method="FP.Close"(reference=w263, error in=w264) -> (error out=w265:errorcluster)  [unwired: 1 in, 2 out]
                      }
                    }
                  }
                }
              }
              frame condition #1 {
              }
            }
            n110 = call <vilib>:"Add State(s) to Queue__jki_lib_state_machine.vi"("State(s) in (\"\")"=w239) -> ("States Out"=w238:string)  [unwired: 14 in]
          }
          frame "UI: Update Graphs" {
            n111 = Unbundle By Name(w271) -> ("IVCurve Data"=w270:cluster{"X":dbl, "Y":dbl}[])
            n112 = property on="I/V Curve" class="XYGraph (strict)"(error in=w267, "Value"=w270) -> (error out=w269:errorcluster)  [unwired: 1 in, 1 out]
            n113 = Merge Errors(w269) -> (w268:errorcluster)
            n114 = call <vilib>:"Add State(s) to Queue__jki_lib_state_machine.vi"("State(s) in (\"\")"=w274) -> ("States Out"=w273:string)  [unwired: 14 in]
          }
          frame "---------- Macro ----------" {
            # "Do not put any code in this frame.\n(It is a separator no-op. You can make a copy of this frame to create a new Macro frame)"
            n115 = call <vilib>:"Add State(s) to Queue__jki_lib_state_machine.vi"("State(s) in (\"\")"=w279) -> ("States Out"=w278:string)  [unwired: 14 in]
          }
          frame "Macro: Initialize" {
            w282 = "UI: Initialize\n//UI: Front Panel State >> Open"  # UI: Initialize //UI: Front Panel State >> Open
            # "Initialization Macro\n(This is called once, when the VI starts)"
            n116 = call <vilib>:"Add State(s) to Queue__jki_lib_state_machine.vi"("State(s) in Front (\"\")"="Data: Initialize\nInitialize Core Data\nEvents: Register", "State(s) in (\"\")"="Process: Sync", "State(s) at Back (\"\")"=w282) -> ("States Out"=w281:string)  [unwired: 12 in]
            n117 = call <vilib>:"Add State(s) to Queue__jki_lib_state_machine.vi"("State(s) in Front (\"\")"=w281, "State(s) in (\"\")"=w288) -> ("States Out"=w287:string)  [unwired: 13 in]
          }
          frame "Macro: Exit" {
            # "Exit Macro\n(This is called once, when the VI exits)"
            n118 = Unbundle By Name(w293) -> ("Core.Close Panel on Exit?"=w299:bool)
            n119 = Select(t="//UI: Front Panel State >> Close", s=w299, f="") -> (s? t:f=w296:string)
            n120 = call <vilib>:"Add State(s) to Queue__jki_lib_state_machine.vi"("State(s) in Front (\"\")"="Data: Cleanup\nEvents: Unregister", "State(s) in (\"\")"="Process: Sync", "State(s) at Back (\"\")"="Exit") -> ("States Out"=w290:string)  [unwired: 12 in]
            n121 = call <vilib>:"Add State(s) to Queue__jki_lib_state_machine.vi"("State(s) in (\"\")"=w296, "State(s) at Back (\"\")"=w290) -> ("States Out"=w295:string)  [unwired: 13 in]
            n122 = call <vilib>:"Add State(s) to Queue__jki_lib_state_machine.vi"("State(s) in Front (\"\")"=w295, "State(s) in (\"\")"=w302) -> ("States Out"=w301:string)  [unwired: 13 in]
          }
          frame "---------- Process ----------" {
            # "Template Separator\n(You can make a copy of, or modify, this frame)"
            n123 = call <vilib>:"Add State(s) to Queue__jki_lib_state_machine.vi"("State(s) in (\"\")"=w307) -> ("States Out"=w306:string)  [unwired: 14 in]
          }
          frame "Process: Sync" {
            n124 = Unbundle By Name(w315) -> ("Self Reference"=w311:refnum<class "Measurement.IVCurve.UI.lvclass">)
            n125 = call <vilib>:"WaitOnProcessSync.vi"("error in (no error)"=w310, "SMO"=w311) -> ("error out"=w309:errorcluster, "Don't run?"=w314:bool)  [unwired: 7 in, 1 out]
            n126 = Select(t="Data: Cleanup\nEvents: Unregister\nExit", s=w314, f="") -> (s? t:f=w308:string)
            n127 = call <vilib>:"Add State(s) to Queue__jki_lib_state_machine.vi"("State(s) in Front (\"\")"=w308, "State(s) in (\"\")"=w318) -> ("States Out"=w317:string)  [unwired: 13 in]
          }
          frame "---------- Events ----------" {
            # "Template Separator\n(You can make a copy of, or modify, this frame)"
            n128 = call <vilib>:"Add State(s) to Queue__jki_lib_state_machine.vi"("State(s) in (\"\")"=w323) -> ("States Out"=w322:string)  [unwired: 14 in]
          }
          frame "Events: Register" {
            # "Measurement base class Public Events"
            # "Base Class Protected Events"
            n129 = Unbundle By Name(w329) -> ("Self Reference"=w334:refnum<class "Measurement.IVCurve.UI.lvclass">)
            n130 = Unbundle By Name(w329) -> ("Dependencies.Measurement.IVCurve"=w328:refnum<class "Measurement.IVCurve.lvclass">)
            n131 = call <vilib>:"GetProtectedEvents.vi"("SMO"=w334) -> ("error out"=w330:errorcluster, "SMO Protected Events"=w335:T12)  [unwired: 8 in, 1 out]
            n132 = call "Measurement.GetPublicEventsRegistration.vi"("Measurement in"=w328) -> ("error out"=w324:errorcluster, "Measurement Public Events"=w325:refnum<event-registration>)  [unwired: 8 in, 1 out]
            n133 = register-events(w335) -> (reference out=w327:refnum<event-registration>, error out=w332:errorcluster)  [unwired: 2 in]
            n134 = Bundle("Event Registration Refnum"=w327, "Measurement Public Events"=w325) -> (w326:T13)  [unwired: 1 in]
            n135 = Merge Errors(w333, w332, w330, w324) -> (w331:errorcluster)
            n136 = call <vilib>:"Add State(s) to Queue__jki_lib_state_machine.vi"("State(s) in (\"\")"=w337) -> ("States Out"=w336:string)  [unwired: 14 in]
          }
          frame "Events: Unregister" {
            n137 = Unregister For Events(event registration refnum=w340, error in=w339) -> (error out=w338:errorcluster)
            n138 = call <vilib>:"Add State(s) to Queue__jki_lib_state_machine.vi"("State(s) in (\"\")"=w343) -> ("States Out"=w342:string)  [unwired: 14 in]
          }
          frame "---------- Action ----------" {
            n139 = Unbundle By Name(w346) -> ("Self Reference"=w344:refnum<class "Measurement.IVCurve.UI.lvclass">)
            n140 = Bundle By Name(cluster=w346, "Self Reference"=w344) -> (w345:T9)
            n141 = call <vilib>:"Add State(s) to Queue__jki_lib_state_machine.vi"("State(s) in (\"\")"=w350) -> ("States Out"=w349:string)  [unwired: 14 in]
          }
          frame "Action: Notify UI Closed" {
            # "Notify that the UI has been closed"
            n142 = Unbundle By Name(w353) -> ("Self Reference"=w354:refnum<class "Measurement.IVCurve.UI.lvclass">)
            n143 = call <vilib>:"Hide.vi"("error in (no error)"=w352, "SMO.UI"=w354) -> ("error out"=w351:errorcluster)  [unwired: 8 in, 1 out]
            n144 = call <vilib>:"Add State(s) to Queue__jki_lib_state_machine.vi"("State(s) in (\"\")"=w357) -> ("States Out"=w356:string)  [unwired: 14 in]
          }
        }
      }
    }
    frame Error {
    }
  }
  n145 = call-parent "Process.vi"("error in (no error)"=w8, "SMO.UI"=w7) -> ("error out"=w5:errorcluster, "SMO.UI out"=→"Measurement.WavelengthSweeping.UI out":refnum<class "Measurement.IVCurve.UI.lvclass">)  [unwired: 8 in]
  n146 = Merge Errors(w5, w4) -> (→"error out":errorcluster)
